vi "2HP_Clone.vi"(0 "Single 2HP":T1) -> (1 "Serial number":u32, 2 "DAQ Error":errorcluster, 3 "All samples out":sgl[][](array[numeric]), 4 "Ch No":i16[](array[numeric]), 5 "Index":i32[](array[numeric]), 6 "Sampling Rate Hz":dbl)   [LabVIEW 2021]
doc: "Use this plug-in with the Nathan 7609 data acquisition system"
uses:
  Device ID port info.ctl
  ctls/2HP_Cmd (USB).ctl
  Globals/Meas_global.vi
  Globals/Extra_Commands_Global.vi
  Globals/Trav_pos_global.vi
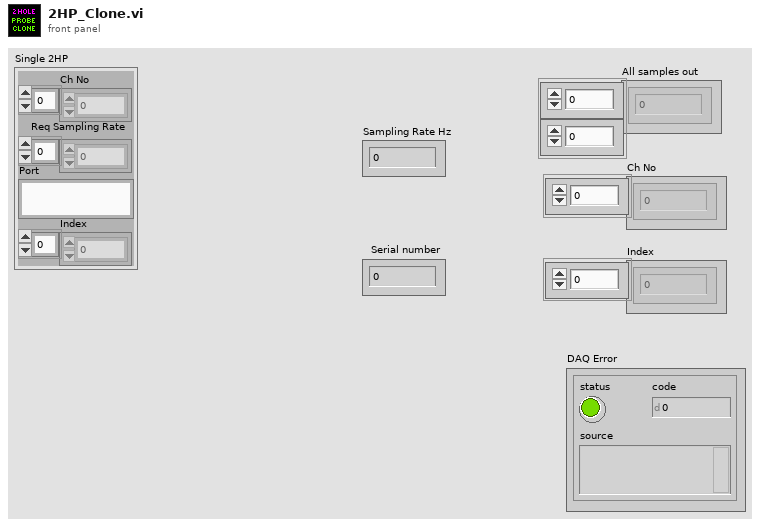
[diagram p1: front panel]
types:
  T1 = typedef "Device ID port info.ctl" = cluster{"Ch No":i16[], "Req Sampling Rate":dbl[], "Port":string, "Index":i32[]}
  T2 = typedef "Traverse_cluster.ctl" = cluster{"Start X":sgl, "Start Y":sgl, "Start Z":sgl, "End X":sgl, "End Y":sgl, "End Z":sgl, "nPoints":i32, "Spacing":T3, "Filename":path, "Tunnel Speed":dbl, "Averaging time (mins)":dbl, "Extra Commands":string, "Carrier_1 Q (l/min)":dbl, "Carrier_2 Q (l/min)":dbl, "Trace Gas Concentration (%)":dbl, "Specific Arguments":string, "Comments":string, "Row No":i32, "Row Type Selector":T4, "EstCompl":string, "Row Duration (mins)":dbl, "nValidPoints":i32, "Meas Setup File":string}
  T3 = typedef "Spacing.ctl" = enum16{"Linear", "Log", "Gauss", "Specified", "N/A"}
  T4 = typedef "Multi_run_mode.ctl" = enum16{"Move Traverse Only", "Set Tunnel Speed Only", "Set Source Only", "Set Measurement Conditions", "Single Measurement", "Vertical Profile", "Lateral Profile", "Longitudinal Profile", "Multi-Axis Profile", "Explore Volume", "Auto Calibrate", "Meas Fast FID Bkgnd", "Check Beam Power", "Scanning Valve Measurement", "Run VI Named:", "Set ADAM Ch", "Wait (minutes)", "Send Message", "Synchronize With:", "Fall Back to this Row", "Turn Off Row Repeating", "Traverse 3D Volume", "Blank Row", "Jump to Fall Back Row"}
  T5 = typedef "Trigger_Mode.ctl" = enum16{"Free Running", "Start on Trigger", "Trigger Every Block", "Trigger Every Sample"}
  T6 = typedef "2HP_Cmd (USB).ctl" = string
  T7 = typedef "Rendezvous RefNum" = refnum<k1>
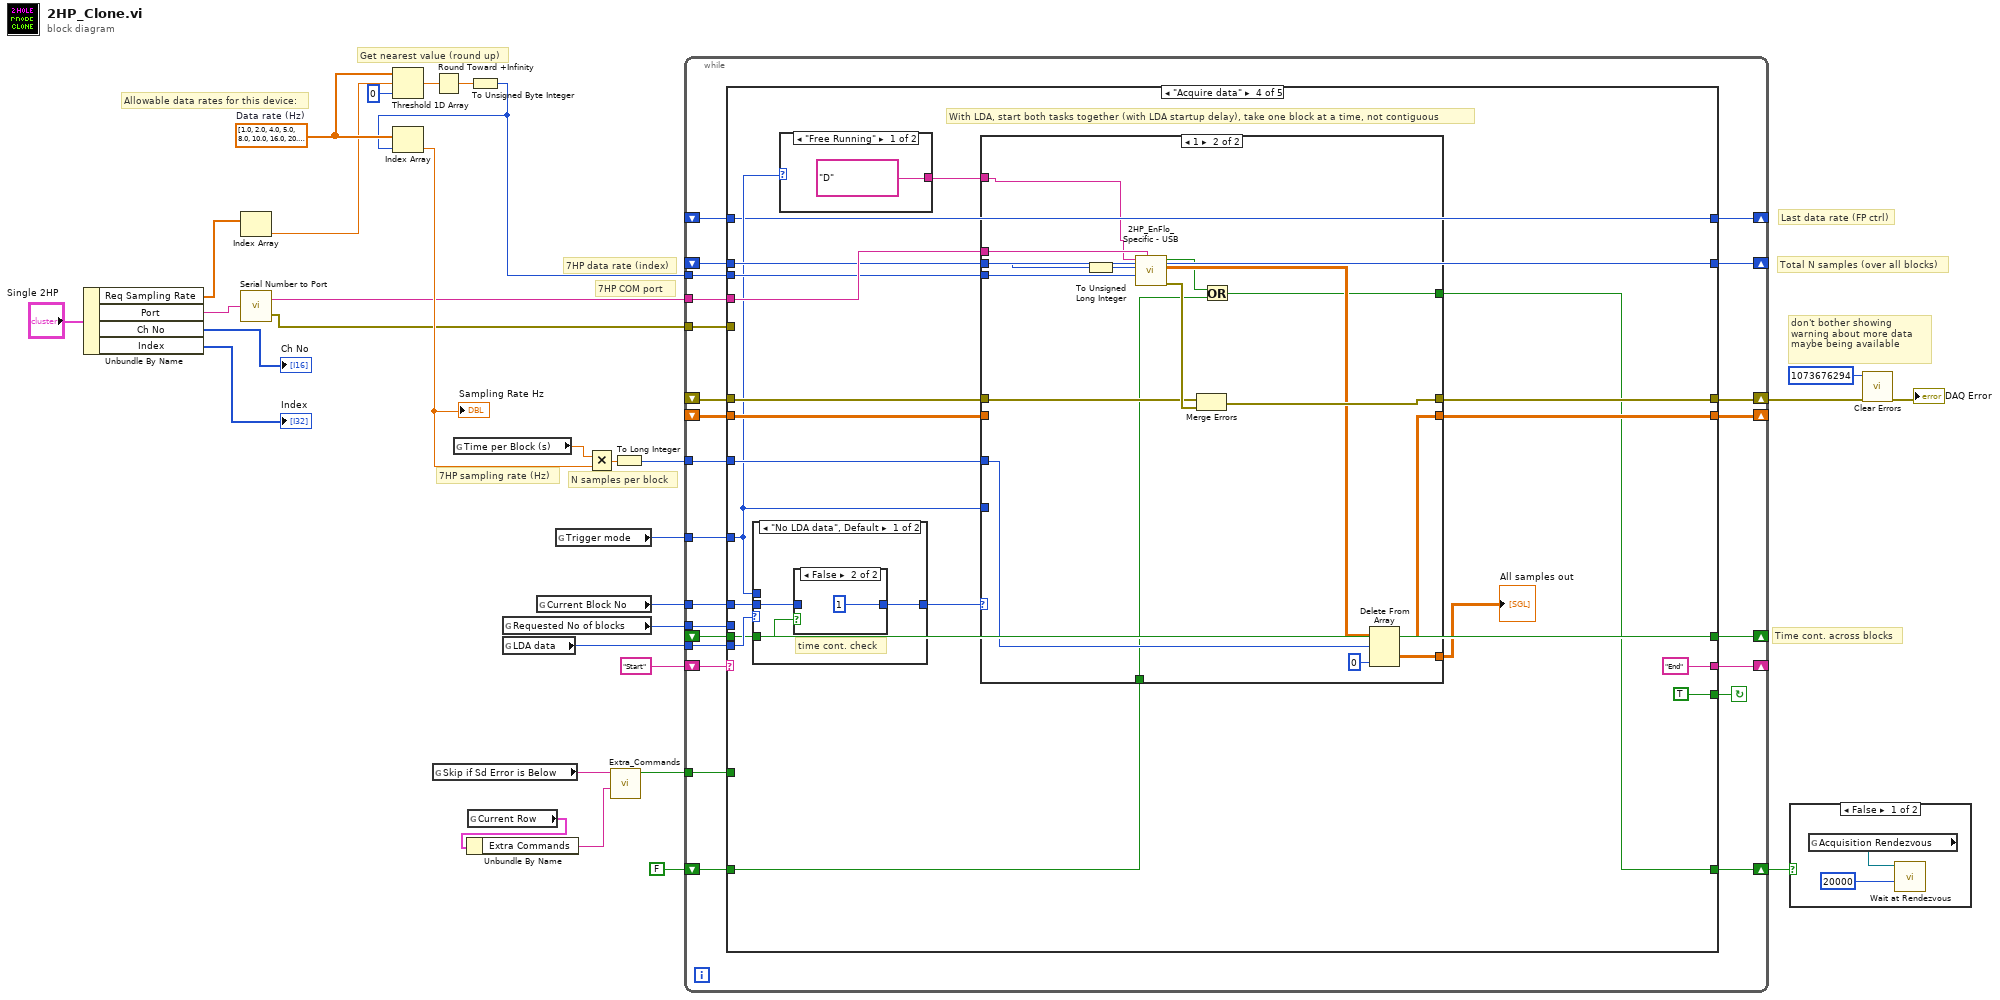
[diagram p0: block diagram]
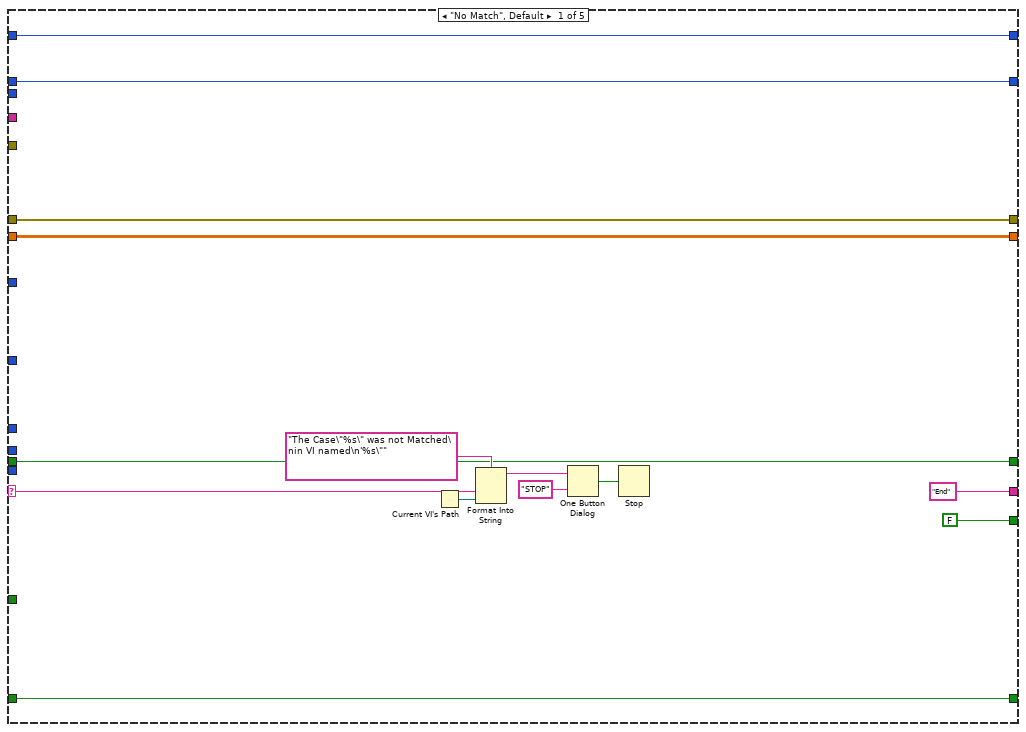
[diagram p3: hidden frame]
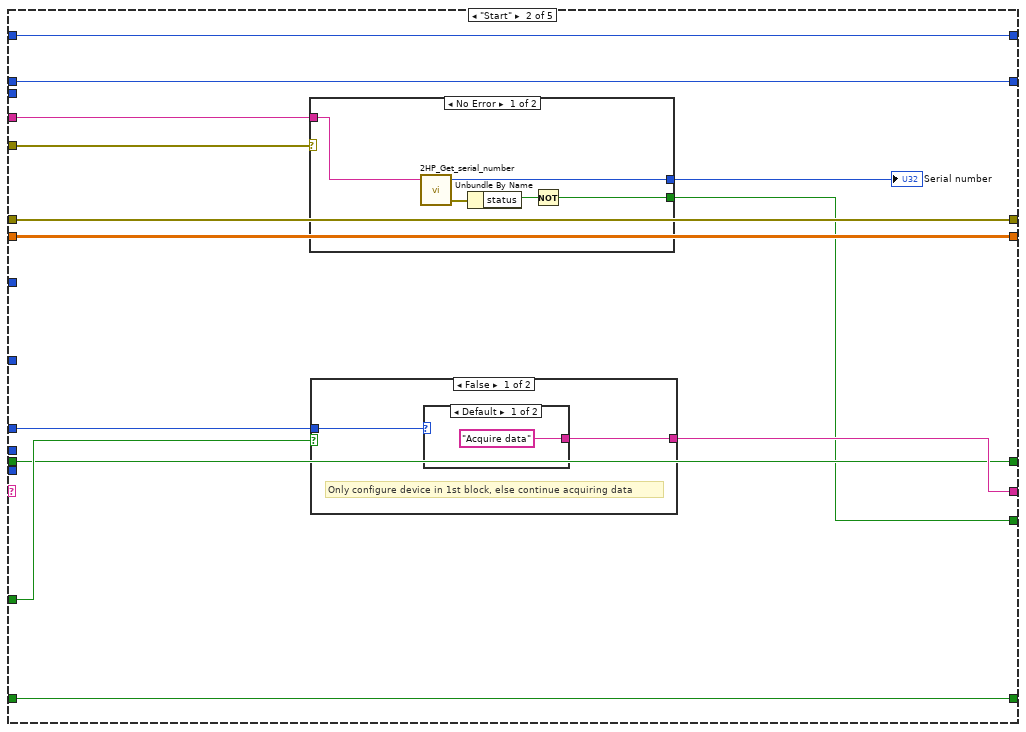
[diagram p4: hidden frame]
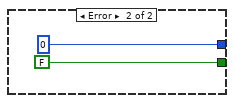
[diagram p5: hidden frame]
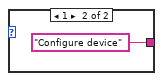
[diagram p6: hidden frame]
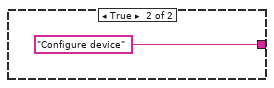
[diagram p7: hidden frame]
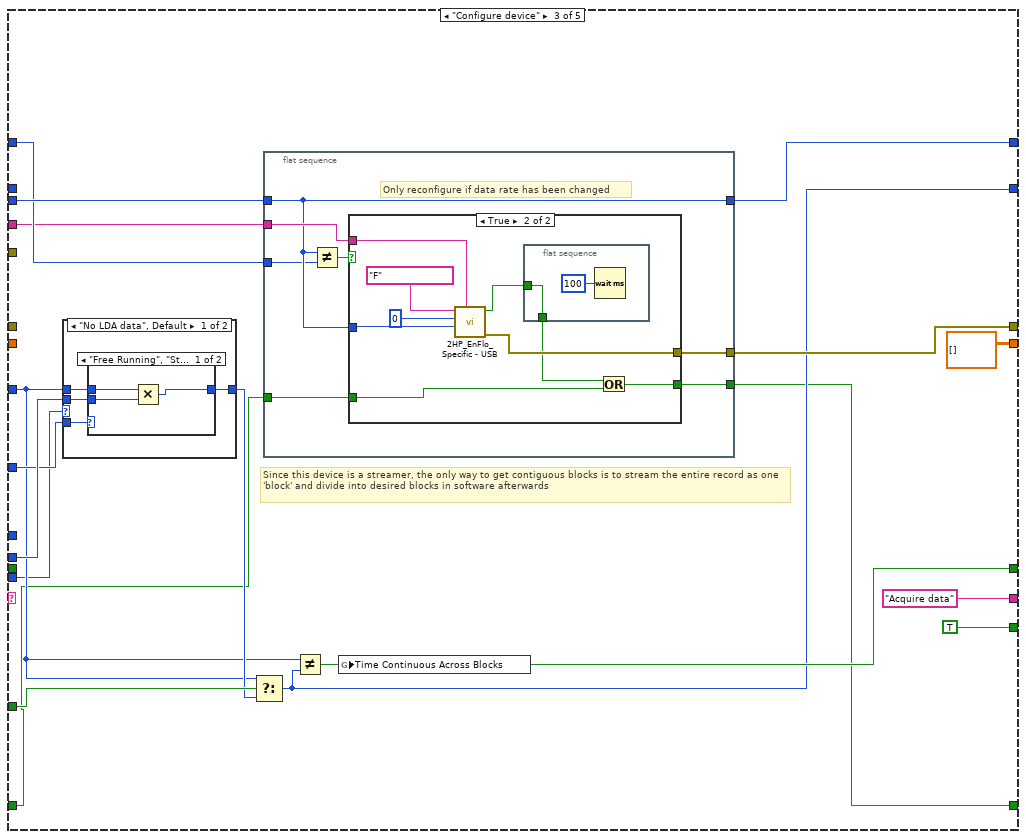
[diagram p8: hidden frame]
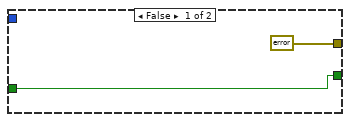
[diagram p11: hidden frame]
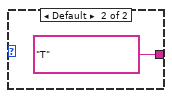
[diagram p12: hidden frame]
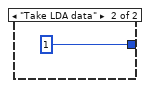
[diagram p14: hidden frame]
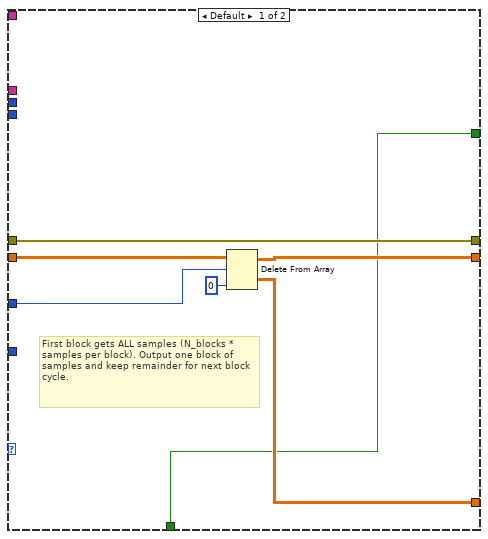
[diagram p15: hidden frame]
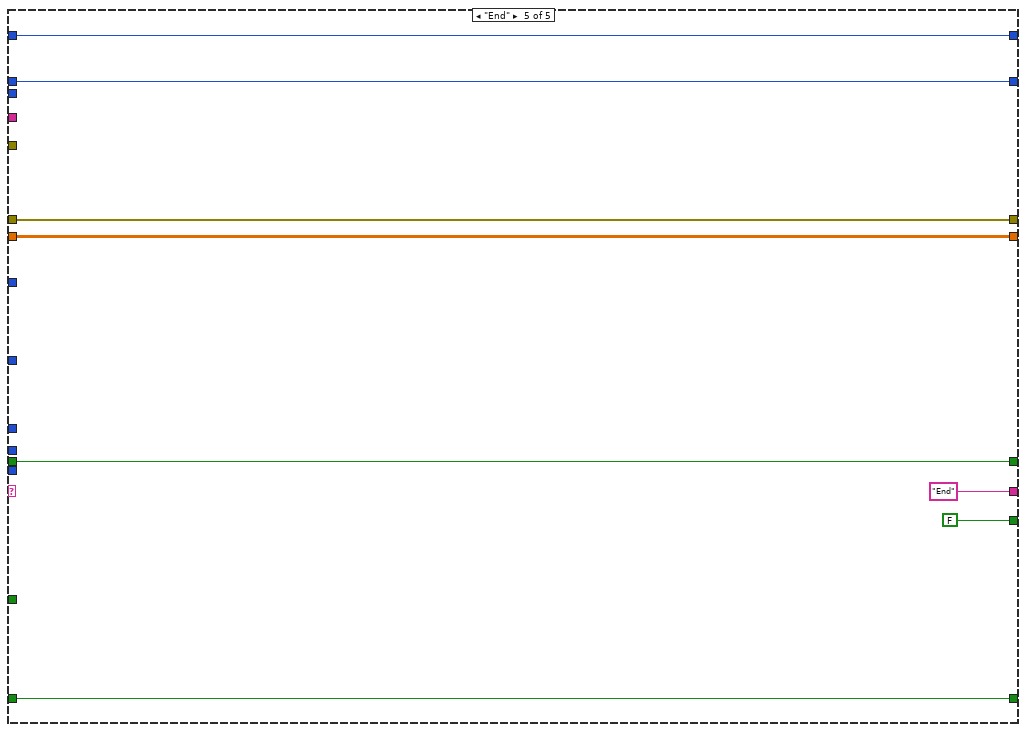
[diagram p16: hidden frame]
diagram:
  w17 = dbl[] [1.0, 2.0, 4.0, 5.0, 8.0, 10.0, 16.0, 20.0, 25.0, 32.0, 40.0, 50.0, 64.0, 80.0, 100.0, 125.0, 160.0, 200.0, 250.0, 320.0, 400.0, 500.0, 625.0, 800.0, 1000.0]  # Data rate (Hz)
  # "N samples per block"
  # "7HP sampling rate (Hz)"
  # "7HP COM port"
  # "7HP data rate (index)"
  # "Allowable data rates for this device:"
  # "Get nearest value (round up)"
  # "Last data rate (FP ctrl)"
  # "Total N samples (over all blocks)"
  # "don't bother showing warning about more data maybe being available"
  # "Time cont. across blocks"
  n1 = Unbundle By Name("Single 2HP") -> ("Req Sampling Rate"=w9:dbl[], "Port"=w3:string, "Ch No"=→"Ch No":i16[], "Index"=→"Index":i32[])
  n2 = Index Array(array=w9) -> (element=w8:dbl)  [unwired: 1 in]
  n3 = call "Serial Number to Port.vi"("Port In"=w3) -> ("Port Out"=w5:string, "error out"=w4:errorcluster)
  n4 = Threshold 1D Array(1:0 ("start index (0)"), 2:w8, 3:w17) -> (0:w18:dbl)
  n5 = global read "Extra_Commands_Global.vi" "Skip if Sd Error is Below"() -> (w25:string)
  n6 = Round Toward +Infinity(x=w18) -> (ceil(x): smallest int >= x=w16:dbl)
  n7 = global read "Meas_global.vi" "Time per Block (s)"() -> (w15:dbl)
  n8 = global read "Trav_pos_global.vi" "Current Row"() -> (w26:T2)
  n9 = Unbundle By Name(w26) -> ("Extra Commands"=w24:string)
  n10 = To Unsigned Byte Integer(number=w16) -> (unsigned 8bit integer=w11:u8)
  n11 = Index Array(array=w17, index=w11) -> (element=w12:dbl)
  "Sampling Rate Hz" <- w12
  n12 = global read "Meas_global.vi" "Requested No of blocks"() -> (w27:i32)
  n13 = global read "Meas_global.vi" "LDA data"() -> (w28:enum16{"No LDA data", "Take LDA data"})
  n14 = global read "Meas_global.vi" "Current Block No"() -> (w29:i32)
  n15 = global read "Meas_global.vi" "Trigger mode"() -> (w30:T5)
  n16 = Multiply(x=w15, y=w12) -> (x*y=w14:dbl)
  n17 = call "Extra_Commands.vi"("String to Search"=w24, "Command"=w25) -> ("Command Found"=w23:bool)  [unwired: 2 in, 3 out]
  n18 = To Long Integer(number=w14) -> (32bit integer=w13:i32)
  n19 = while {
    shift-left: "Start" -> [w55]
    shift-right: [w44] -> _
    tunnel: w13 -> [w54]
    tunnel: w29 -> [w53]
    tunnel: w30 -> [w51]
    tunnel: w28 -> [w50]
    tunnel: w27 -> [w49]
    shift-right: [w47] -> w20
    shift-left: _ -> [w48]
    shift-right: [w46] -> _
    shift-left: _ -> [w45]
    tunnel: w23 -> [w43]
    shift-right: [w42] -> _
    shift-left: _ -> [w41]
    tunnel: w5 -> [w40]
    tunnel: w11 -> [w39]
    shift-right: [w38] -> _
    shift-left: _ -> [w37]
    shift-right: [w36] -> _
    shift-left: _ -> [w35]
    tunnel: w4 -> [w34]
    shift-right: [w33] -> w1
    shift-left: FALSE -> [w32]
    stop <- w52 continue-if-true
    n20 = case shown="\"Acquire data\"" w55 {
      selector: w55 -> [w62 _ _ _ _]
      tunnel: ["End" w80 "Acquire data" ("f") "End" "End" ("f")] -> w44
      tunnel: w54 -> [_ _ w104 w151 _]
      tunnel: w53 -> [_ w81 _ w155 _]
      tunnel: [FALSE w71 TRUE TRUE FALSE] -> w52
      tunnel: w51 -> [_ _ w107 w146 _]
      tunnel: w50 -> [_ _ w102 w154 _]
      tunnel: w49 -> [_ _ w111 _ _]
      tunnel: w48 -> [w61 w82 _ w159 w196]
      tunnel: [w61 w82 w110 w152 w196] -> w47
      tunnel: [w60 w79 sgl[][] [] ("Channel volts") w157 w198] -> w46
      tunnel: w45 -> [w60 w79 _ w158 w198]
      tunnel: w43 -> [_ w78 w106 _ _]
      tunnel: [w59 w77 w103 w153 w197] -> w42
      tunnel: w41 -> [w59 w77 _ w153 w197]
      tunnel: w40 -> [_ w73 w97 w150 _]
      tunnel: w39 -> [_ _ w101 w149 _]
      tunnel: [w57 w75 w100 w148 w194] -> w38
      tunnel: w37 -> [w57 w75 _ w148 w194]
      tunnel: [w58 w76 w99 w144 w195] -> w36
      tunnel: w35 -> [w58 w76 w98 w144 w195]
      tunnel: w34 -> [_ w74 _ _ _]
      tunnel: [w56 w70 w95 w142 w193] -> w33
      tunnel: w32 -> [w56 w70 w96 w143 w193]
      frame "No Match", Default {
        n21 = Current VI's Path() -> (path=w65:path)
        n22 = Format Into String(format string="The Case\"%s\" was not Matched\nin VI named\n'%s\"" ("Format String"), w62, w65) -> (resulting string=w68:string)  [unwired: 2 in, 1 out]
        n23 = One Button Dialog(message=w68, button name ("OK")="STOP") -> (true=w66:bool)
        n24 = Stop(stop? (T)=w66) -> ()
      }
      frame "Start" {
        n25 = case shown="No Error" w74 {
          tunnel: w73 -> [w87 _]
          tunnel: [w86 u32 0 ("Serial number")] -> w72
          tunnel: [w83 FALSE] -> w71
          frame No Error {
            n26 = call "2HP_Get_serial_number.vi"("Port"=w87) -> ("Error Out"=w85:errorcluster, "Serial number"=w86:u32)  [unwired: 3 in]
            n27 = Unbundle By Name(w85) -> ("status"=w84:bool)
            n28 = Not(x=w84) -> (.not. x?=w83:bool)
          }
          frame Error {
          }
        }
        "Serial number" <- w72
        n29 = case shown="False" w78 {
          tunnel: w81 -> [w91 _]
          tunnel: [w90 "Configure device" ("f")] -> w80
          frame False {
            # "Only configure device in 1st block, else continue acquiring data"
            n30 = case shown="Default" w91 {
              tunnel: ["Acquire data" ("f") "Configure device" ("f")] -> w90
              frame Default {
              }
              frame 1 {
              }
            }
          }
          frame True {
          }
        }
      }
      frame "Configure device" {
        # "Since this device is a streamer, the only way to get contiguous blocks is to stream the entire record as one 'block' and divide into desired blocks in software afterwards"
        n31 = case shown="\"No LDA data\", Default" w102 {
          tunnel: [w114 w121] -> w105
          tunnel: w104 -> [w116 w121]
          tunnel: w111 -> [w115 _]
          tunnel: w107 -> [w113 _]
          frame "No LDA data", Default {
            n32 = case shown="\"Free Running\", \"Start on Trigger\"" w113 {
              tunnel: w116 -> [w119 w120]
              tunnel: w115 -> [w118 _]
              tunnel: [w117 w120] -> w114
              frame "Free Running", "Start on Trigger" {
                n33 = Multiply(x=w119, y=w118) -> (x*y=w117:i32)
              }
              frame "Trigger Every Block", Default {
              }
            }
          }
          frame "Take LDA data" {
          }
        }
        n34 = Select(t=w104, s=w106, f=w105) -> (s? t:f=w100:i32)
        n35 = flat-sequence {
          tunnel: [w128] -> w110
          tunnel: w97 -> [w127]
          tunnel: w101 -> [w125]
          tunnel: [w125] -> w99
          tunnel: w98 -> [w124]
          tunnel: w96 -> [w123]
          tunnel: [w122] -> w95
          frame #0 {
            # "Only reconfigure if data rate has been changed"
            n36 = Not Equal?(x=w125, y=w124) -> (x != y?=w126:bool)
            n37 = case shown="True" w126 {
              tunnel: [errorcluster {"status"=FALSE, "code"=0, "source"=""} ("error IO") w136] -> w128
              tunnel: w127 -> [_ w135]
              tunnel: w125 -> [_ w137]
              tunnel: w123 -> [w129 w134]
              tunnel: [w129 w133] -> w122
              frame False {
              }
              frame True {
                n38 = call "2HP_EnFlo_Specific - USB.vi"("COM port"=w135, "Set data rate (Hz)"=w137, "N samples"=u32 0, "Command"=T6 "F") -> ("Error"=w136:errorcluster, "Rendezvous out"=w131:bool)  [unwired: 4 in, 1 out]
                n39 = flat-sequence {
                  tunnel: [w140] -> w132
                  tunnel: w131 -> [w140]
                  frame #0 {
                    n40 = Wait (ms)(milliseconds to wait=u32 100) -> ()  [unwired: 1 out]
                  }
                }
                n41 = Or(x=w132, y=w134) -> (x .or. y?=w133:bool)
              }
            }
          }
        }
        n42 = Not Equal?(x=w104, y=w100) -> (x != y?=w103:bool)
        n43 = global write "Meas_global.vi" "Time Continuous Across Blocks"(w103) -> ()
      }
      frame "Acquire data" {
        # "With LDA, start both tasks together (with LDA startup delay), take one block at a time, not contiguous"
        n44 = case shown="\"No LDA data\", Default" w154 {
          tunnel: w155 -> [w165 _]
          tunnel: w146 -> [_ _]
          tunnel: [w166 1 ("Current Block No")] -> w156
          tunnel: w153 -> [w164 _]
          frame "No LDA data", Default {
            # "time cont. check"
            n45 = case shown="False" w164 {
              tunnel: [w167 1 ("Current Block No")] -> w166
              tunnel: w165 -> [w167 _]
              frame True {
              }
              frame False {
              }
            }
          }
          frame "Take LDA data" {
          }
        }
        n46 = case shown="\"Free Running\"" w146 {
          tunnel: [T6 "D" ("Command") T6 "T" ("Command")] -> w147
          frame "Free Running" {
          }
          frame Default {
          }
        }
        n47 = case shown="1" w156 {
          tunnel: w159 -> [w172 w191]
          tunnel: [w172 w190] -> w152
          tunnel: [w174 w187] -> w157
          tunnel: w151 -> [w173 w188]
          tunnel: w158 -> [w175 _]
          tunnel: [w171 w185] -> w145
          tunnel: w146 -> [_ _]
          tunnel: w150 -> [_ w184]
          tunnel: w149 -> [_ w183]
          tunnel: w148 -> [_ w182]
          tunnel: w147 -> [_ w177]
          tunnel: w143 -> [w170 w179]
          tunnel: [w170 w178] -> w142
          frame Default {
            # "First block gets ALL samples (N_blocks * samples per block). Output one block of samples and keep remainder for next block cycle."
            n48 = Delete From Array(array=w175, length=w173, index (col)=0 ("disabled index (col)")) -> (deleted portion=w171:sgl[][], array with subset deleted=w174:sgl[][])  [unwired: 1 in]
          }
          frame 1 {
            n49 = To Unsigned Long Integer(number=w182) -> (unsigned 32bit integer=w181:u32)
            n50 = call "2HP_EnFlo_Specific - USB.vi"("COM port"=w184, "Set data rate (Hz)"=w183, "N samples"=w181, "Command"=w177) -> ("Error"=w192:errorcluster, "All samples out"=w189:sgl[][], "Rendezvous out"=w180:bool)  [unwired: 4 in]
            n51 = Merge Errors(w191, w192) -> (w190:errorcluster)
            n52 = Or(x=w180, y=w179) -> (x .or. y?=w178:bool)
            n53 = Delete From Array(array=w189, length=w188, index (col)=0 ("disabled index (col)")) -> (deleted portion=w185:sgl[][], array with subset deleted=w187:sgl[][])  [unwired: 1 in]
          }
        }
        "All samples out" <- w145
      }
      frame "End" {
      }
    }
  }
  n54 = case shown="False" w1 {
    frame False {
      n55 = global read "Meas_global.vi" "Acquisition Rendezvous"() -> (w202:T7)
      n56 = call <vilib>:"Wait at Rendezvous.vi"("ms timeout (-1)"=20000, "rendezvous"=w202) -> ()  [unwired: 3 in, 3 out]
    }
    frame True {
    }
  }
  n57 = call <vilib>:"Clear Errors.vi"("error in (no error)"=w20, "specific error code to clear (0: all)"=1073676294) -> ("error out"=→"DAQ Error":errorcluster)  [unwired: 4 in, 1 out]
